vi "Two Gaussians Fit Guess Parameters.vi"(8 "Cursor X 2":dbl, 9 "Cursor X 1":dbl, 10 "Y Array":dbl[](array[numeric]), 11 "X Array":dbl[](array[numeric])) -> (1 "Guess Parameters Array":dbl[](array[numeric]), 2 "Y Array dup":dbl[](array[numeric]), 3 "X Array dup":dbl[](array[numeric]))   [LabVIEW 2021, in "Fits.lvlib"]
uses:
  Fits.lvlib
  Histograms/Histogram Window.lvlib
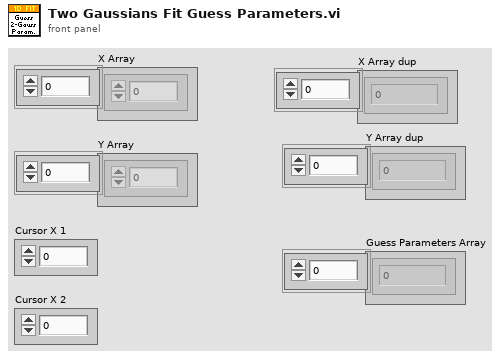
[diagram p1: front panel]
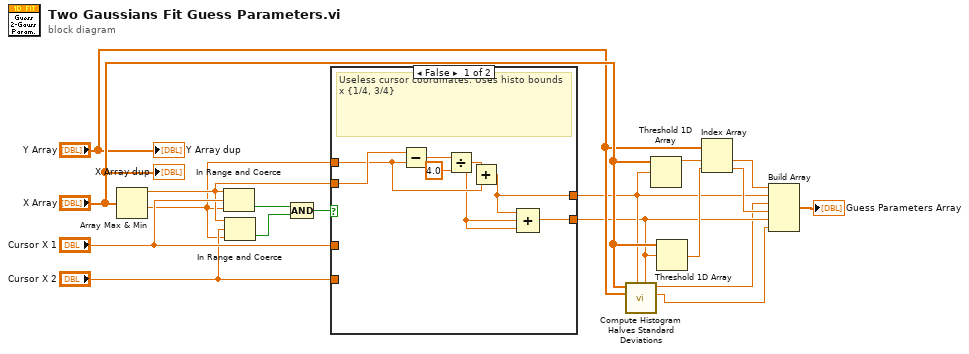
[diagram p0: block diagram]
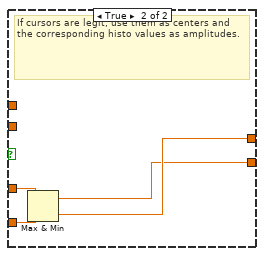
[diagram p2: hidden frame]
diagram:
  n1 = Array Max & Min(array="X Array") -> (max value=w11:dbl, min value=w10:dbl)  [unwired: 2 out]
  n2 = In Range and Coerce(upper limit=w11, x="Cursor X 1", lower limit=w10) -> (In Range?=w18:bool)  [unwired: 1 out]
  n3 = In Range and Coerce(upper limit=w11, x="Cursor X 2", lower limit=w10) -> (In Range?=w17:bool)  [unwired: 1 out]
  n4 = Compound Arithmetic op=AND(w18, w17) -> (w16:bool)
  n5 = case shown="False" w16 {
    tunnel: "Cursor X 1" -> [_ w29]
    tunnel: "Cursor X 2" -> [_ w28]
    tunnel: [w21 w27] -> w4
    tunnel: [w19 w26] -> w3
    tunnel: w11 -> [w23 _]
    tunnel: w10 -> [w22 _]
    frame False {
      # "Useless cursor coordinates. Uses histo bounds x {1/4, 3/4}"
      n6 = Subtract(x=w23, y=w22) -> (x-y=w25:dbl)
      n7 = Divide(x=w25, y=4.0) -> (x/y=w20:dbl)
      n8 = Add(x=w20, y=w22) -> (x+y=w21:dbl)
      n9 = Compound Arithmetic op=ADD(w21, w20, w20) -> (w19:dbl)
    }
    frame True {
      # "If cursors are legit, use them as centers and the corresponding histo values as amplitudes."
      n10 = Max & Min(x=w29, y=w28) -> (max(x,y)=w26:dbl, min(x,y)=w27:dbl)
    }
  }
  n11 = call "Compute Histogram Halves Standard Deviations.vi"("x 2"=w3, "x 1"=w4, "Y Array"="Y Array", "X Array"="X Array") -> ("SDV 2"=w1:dbl, "SDV 1"=w2:dbl)  [unwired: 5 in, 1 out]
  n12 = Threshold 1D Array(2:w4, 3:"X Array") -> (0:w12:dbl)  [unwired: 1 in]
  n13 = Threshold 1D Array(2:w3, 3:"X Array") -> (0:w8:dbl)  [unwired: 1 in]
  n14 = Index Array(array="Y Array", index #1=w12, index #2=w8) -> (element #1=w13:dbl, element #2=w7:dbl)
  n15 = Build Array(w13, w4, w2, w7, w3, w1) -> (→"Guess Parameters Array":dbl[])
  "X Array dup" <- "X Array"
  "Y Array dup" <- "Y Array"
